vi "Start Chassis.vi"(5 "Cfg wChassis":T1, 6 "Show FP?":bool, 7 "Actor-to-Caller Enqueuer":refnum<class "Message Enqueuer.lvclass">, 8 "error in":errorcluster, 9 "TCP LS Writer":refnum<class "Message Enqueuer.lvclass">, 10 "TCP HS Writer":refnum<class "Message Enqueuer.lvclass">, 11 "Master Slave":refnum<class "Master Slave.lvclass">) -> (0 "error out":errorcluster, 3 "Master Slave":refnum<class "Master Slave.lvclass">)   [LabVIEW 2012, in "Data Acquisition.lvlib" / "Master Slave.lvclass"]
uses:
  Master Slave.lvclass
  <vilib>/ActorFramework/Message Enqueuer/Message Enqueuer.lvclass
  Custom Ctrls/Master Cfg/ge_Cfg wChassis.ctl
  Cfg Grandmaster/Class Chassis BOM/Chassis BOM.lvclass
  Cfg Grandmaster/Class Chassis Cfg/ChassisCfg.lvclass
  Class Chassis Tasks/Chassis Tasks.lvclass
  Common/Controls/TE_Designator.ctl
  Class DAQ Actor/DAQ Actor.lvclass
  Class DAQ Actor Slave/DAQ Actor (Slave).lvclass
  Class Chassis Tasks/Chassis Tasks.lvclass/Chassis Tasks.ctl
  <vilib>/ActorFramework/Message Enqueuer/Message Enqueuer.lvclass/Message Enqueuer.ctl
  Class Chassis Tasks/Read LS DAQ Task.vi
  Class Chassis Tasks/Read HS DAQ Task.vi
  Class Chassis Tasks/Write LS ActorQ.vi
  Class Chassis Tasks/Write HS ActorQ.vi
  <vilib>/ActorFramework/Message Enqueuer/Enqueue.vi
  <vilib>/ActorFramework/Message Priority Queue/Priority Enqueue.vi
  Class DAQ Task/DAQ Task.lvclass
  DAQ Actor Messages/Start Task Msg/Start Task Msg.lvclass
  <vilib>/ActorFramework/Actor/Actor.lvclass
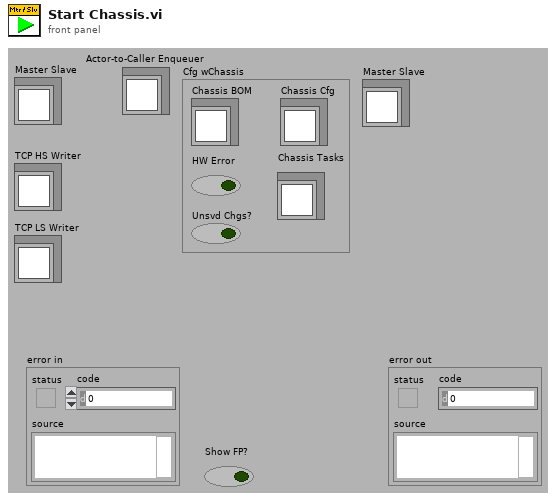
[diagram p1: front panel]
types:
  T1 = typedef "ge_Cfg wChassis.ctl" = cluster{"Chassis BOM":refnum<class "Chassis BOM.lvclass">, "Chassis Cfg":refnum<class "ChassisCfg.lvclass">, "Chassis Tasks":refnum<class "Chassis Tasks.lvclass">, "HW Error":bool, "Unsvd Chgs?":bool}
  T2 = typedef "TE_Designator.ctl" = enum16{"High Speed", "Low Speed"}
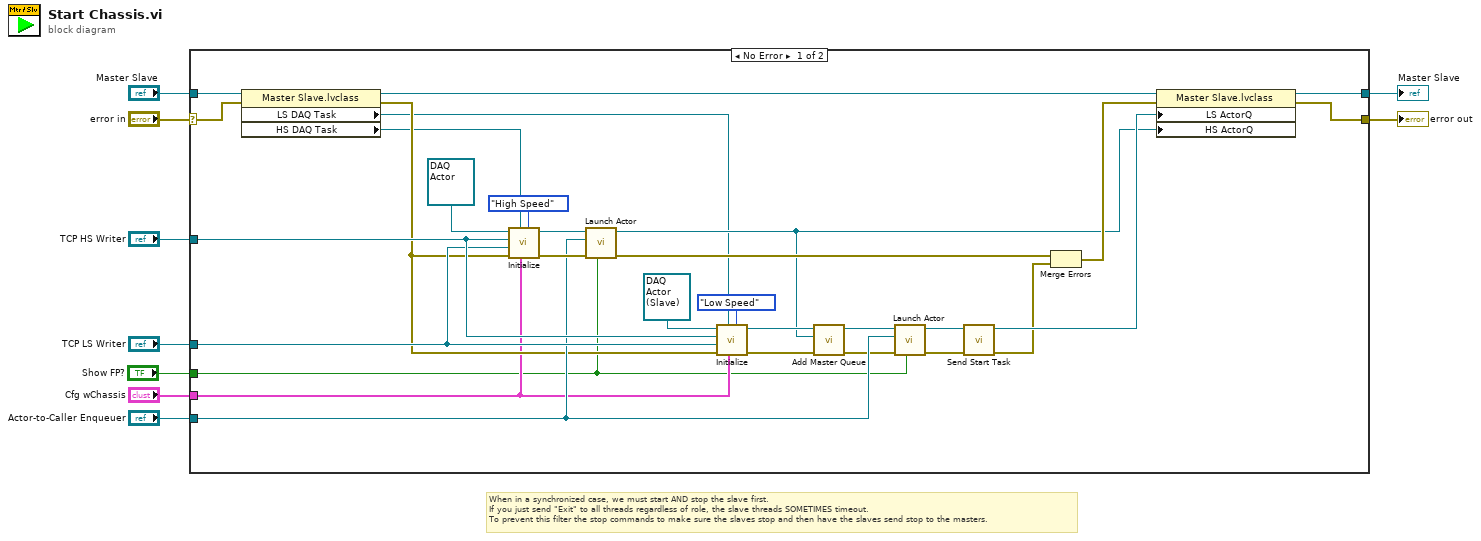
[diagram p0: block diagram]
diagram:
  # "When in a synchronized case, we must start AND stop the slave first.\nIf you just send \"Exit\" to all threads regardless of role, the slave threads SOMETIMES timeout.\nTo prevent this filter the stop commands to make sure the slaves stop and then have the slaves send stop to the masters."
  n1 = case shown="No Error" "error in" {
    selector: "error in" -> [w27 w41]
    tunnel: "Master Slave" -> [w35 w40]
    tunnel: "Cfg wChassis" -> [w13 _]
    tunnel: "TCP HS Writer" -> [w34 _]
    tunnel: "TCP LS Writer" -> [w33 _]
    tunnel: "Actor-to-Caller Enqueuer" -> [w23 _]
    tunnel: [w31 w41] -> w4
    tunnel: [w30 w40] -> w3
    tunnel: "Show FP?" -> [w10 _]
    frame No Error {
      n2 = property class="Master Slave.lvclass"(reference=w35, error in=w27) -> (reference out=w32:refnum<class "Master Slave.lvclass">, error out=w16:errorcluster, "LS DAQ Task"=w14:refnum<class "DAQ Task.lvclass">, "HS DAQ Task"=w15:refnum<class "DAQ Task.lvclass">)
      n3 = call-dynamic "Initialize.vi"("TimingEngine"=TE_Designator."High Speed", "Cfg wChassis"=w13, "LS DAQ Task"=w15, "error in (no error)"=w16, "TCP LS Writer"=w33, "TCP HS Writer"=w34, "DAQ Actor in"=refnum<class "DAQ Actor.lvclass"> refnum) -> ("error out"=w37:errorcluster, "DAQ Actor out"=w36:refnum<class "DAQ Actor.lvclass">)  [unwired: 3 in]
      n4 = call <vilib>:"Launch Actor.vi"("Open Actor Core front panel? (F)"=w10, "error in (no error)"=w37, "Actor-to-Caller Enqueuer"=w23, "Actor"=w36) -> ("error out"=w22:errorcluster, "Caller-To-Actor Enqueuer"=w17:refnum<class "Message Enqueuer.lvclass">)  [unwired: 6 in]
      n5 = call-dynamic "Initialize.vi"("TimingEngine"=TE_Designator."Low Speed", "Cfg wChassis"=w13, "LS DAQ Task"=w14, "error in (no error)"=w16, "TCP LS Writer"=w33, "TCP HS Writer"=w34, "DAQ Actor in"=refnum<class "DAQ Actor (Slave).lvclass"> refnum ("Data Acquisition.lvlib:DAQ Actor (Slave).lvclass")) -> ("error out"=w20:errorcluster, "DAQ Actor out"=w21:refnum<class "DAQ Actor (Slave).lvclass">)  [unwired: 3 in]
      n6 = call "Add Master Queue.vi"("error in (no error)"=w20, "Master Actor Q"=w17, "DAQ Actor (Slave)"=w21) -> ("error out"=w18:errorcluster, "DAQ Actor (Slave) out"=w19:refnum<class "DAQ Actor (Slave).lvclass">)  [unwired: 7 in]
      n7 = call <vilib>:"Launch Actor.vi"("Open Actor Core front panel? (F)"=w10, "error in (no error)"=w18, "Actor-to-Caller Enqueuer"=w23, "Actor"=w19) -> ("error out"=w28:errorcluster, "Caller-To-Actor Enqueuer"=w29:refnum<class "Message Enqueuer.lvclass">)  [unwired: 6 in]
      n8 = call "Send Start Task.vi"("error in (no error)"=w28, "Message Enqueuer"=w29) -> ("error out"=w25:errorcluster, "Message Enqueuer out"=w26:refnum<class "Message Enqueuer.lvclass">)  [unwired: 8 in]
      n9 = Merge Errors(w22, w25) -> (w24:errorcluster)
      n10 = property class="Master Slave.lvclass"(reference=w32, error in=w24, "LS ActorQ"=w26, "HS ActorQ"=w17) -> (reference out=w30:refnum<class "Master Slave.lvclass">, error out=w31:errorcluster)
    }
    frame Error {
    }
  }
  "error out" <- w4
  "Master Slave" <- w3
